vi "Func-Math-Extractor.vi"(10 "Fn Math":string[](array[string]), 11 "Fn Arg Cnt":string[](array[string])) -> (2 "Fn-Math":string[](array[string]))   [LabVIEW 2014]
doc: "This VI extracts the math of a function."
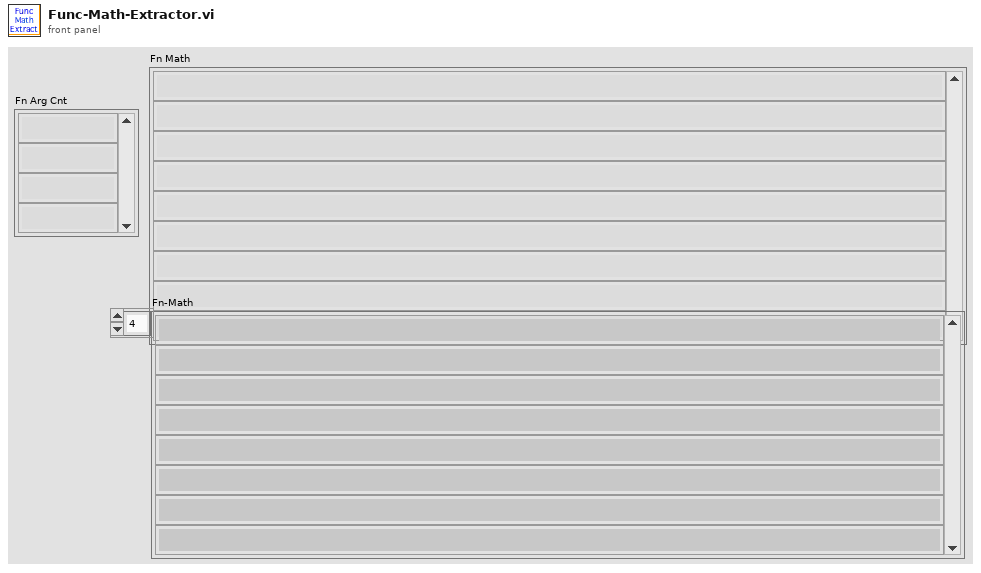
[diagram p1: front panel]
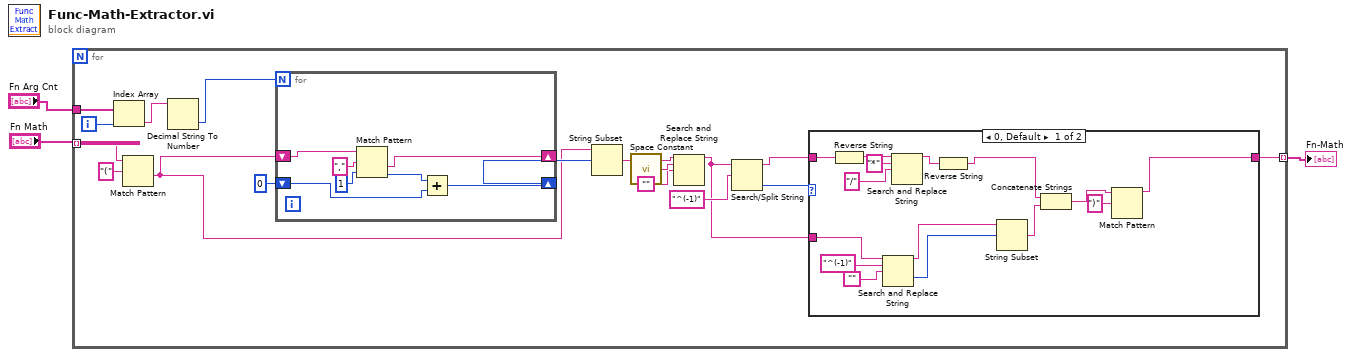
[diagram p0: block diagram]
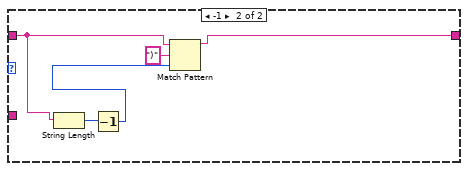
[diagram p2: hidden frame]
diagram:
  n1 = for {
    tunnel: "Fn Math" -> [w6] mode=indexing
    tunnel: [w15] -> w2 mode=indexing
    tunnel: "Fn Arg Cnt" -> [w9]
    i -> [w10]
    n2 = Index Array(array=w9, index=w10) -> (element=w8:string)
    n3 = Match Pattern(string=w6, regular expression="(") -> (after substring=w4:string)  [unwired: 1 in, 3 out]
    n4 = Decimal String To Number(string=w8) -> (number=w7:i32)  [unwired: 2 in, 1 out]
    n5 = for {
      N: w7 -> [_]
      shift-right: [w41] -> _
      shift-left: w4 -> [w47]
      shift-right: [w44] -> w19
      shift-left: 0 -> [w42]
      n6 = Match Pattern(string=w47, regular expression="," ("search string/char (-)"), offset (0)=1) -> (after substring=w41:string, offset past match=w43:i32)  [unwired: 2 out]
      n7 = Add(x=w43, y=w42) -> (x+y=w44:i32)
    }
    n8 = String Subset(string=w4, offset (0)=w19) -> (substring=w18:string)  [unwired: 1 in]
    n9 = call <vilib>:"Space Constant.vi"() -> ("String"=w17:string)
    n10 = Search and Replace String(input string=w18, search string=w17, replace string="") -> (result string=w11:string)  [unwired: 5 in, 3 out]
    n11 = Search/Split String(string=w11, search string/char (-)="^(-1)" ("regular expression")) -> (substring before match=w13:string, offset of match=w12:i32)  [unwired: 1 in, 1 out]
    n12 = case shown="0, Default" w12 {
      tunnel: [w22 w39] -> w15
      tunnel: w13 -> [w29 w38]
      tunnel: w11 -> [w28 _]
      frame 0, Default {
        n13 = Reverse String(1:w29) -> (0:w34:string)
        n14 = Search and Replace String(input string=w28, search string="^(-1)" ("regular expression"), replace string="") -> (result string=w21:string, offset past replacement=w27:i32)  [unwired: 5 in, 2 out]
        n15 = Search and Replace String(input string=w34, search string="*", replace string="/" ("replace string (\"\")")) -> (result string=w31:string)  [unwired: 5 in, 3 out]
        n16 = Reverse String(1:w31) -> (0:w24:string)
        n17 = String Subset(string=w21, offset (0)=w27) -> (substring=w25:string)  [unwired: 1 in]
        n18 = Concatenate Strings(w24, w25) -> (w23:string)
        n19 = Match Pattern(string=w23, regular expression=")") -> (before substring=w22:string)  [unwired: 1 in, 3 out]
      }
      frame -1 {
        n20 = String Length(string=w38) -> (length=w37:i32)
        n21 = Decrement(x=w37) -> (x-1=w36:i32)
        n22 = Match Pattern(string=w38, regular expression=")", offset (0)=w36) -> (before substring=w39:string)  [unwired: 3 out]
      }
    }
  }
  "Fn-Math" <- w2
